vi "ServiceLocationPool_GetLocation_ReturnsValidLocation.vi"(8 "error in (no error)":errorcluster) -> (0 "error out":errorcluster, 2 "result":string, 3 "pass":bool)   [LabVIEW 2020, in "MeasurementServerTests.lvlib"]
uses:
  MeasurementServerTests.lvlib
  Runtime/MeasurementLink Discovery Client/RPC Messages/ni_measurementlink_discovery_v1_ResolveServiceRequest.ctl
  Runtime/MeasurementLink Measurement Server/MeasurementLink Measurement Server.lvlib
  Runtime/MeasurementLink Discovery Client/MeasurementLink Discovery Client.lvlib
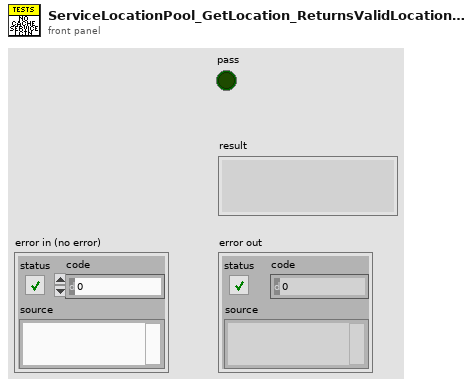
[diagram p1: front panel]
types:
  T1 = typedef "MeasurementLink Discovery Client.lvlib/ni_measurementlink_discovery_v1_ResolveServiceRequest.ctl" = cluster{"provided_interface":string, "service_class":string}
  T2 = typedef "MeasurementLink Discovery Client.lvlib/ni_measurementlink_discovery_v1_ServiceLocation.ctl" = cluster{"location":string, "insecure_port":string, "ssl_authenticated_port":string}
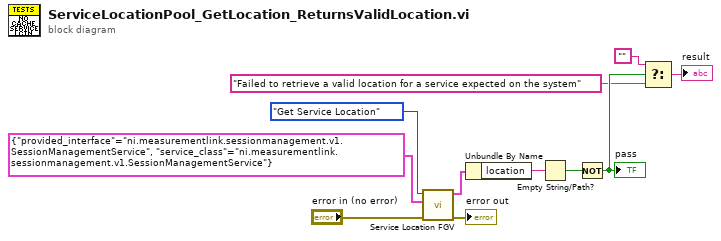
[diagram p0: block diagram]
diagram:
  n1 = call "Service Location FGV.vi"("error in"="error in (no error)", "Resolve Service Request"=T1 {"provided_interface"="ni.measurementlink.sessionmanagement.v1.SessionManagementService", "service_class"="ni.measurementlink.sessionmanagement.v1.SessionManagementService"}, "Action"=enum16{"Get Service Location", "Clear Cache"}."Get Service Location") -> ("error out"=→"error out":errorcluster, "Service Location"=w7:T2)  [unwired: 7 in]
  n2 = Unbundle By Name(w7) -> ("location"=w6:string)
  n3 = Empty String/Path?(string/path=w6) -> (empty?=w5:bool)
  n4 = Not(x=w5) -> (.not. x?=w3:bool)
  "pass" <- w3
  n5 = Select(t="", s=w3, f="Failed to retrieve a valid location for a service expected on the system") -> (s? t:f=→"result":string)
